vi "Message.vi"(8 "error in (no error)":errorcluster, 9 "Additional text":string, 10 "Message":T1) -> (0 "error out":errorcluster)   [LabVIEW 2013, in "Template-class-by-reference.lvlib" / "Template.lvclass"]
uses:
  Template.lvclass
  Messages.ctl
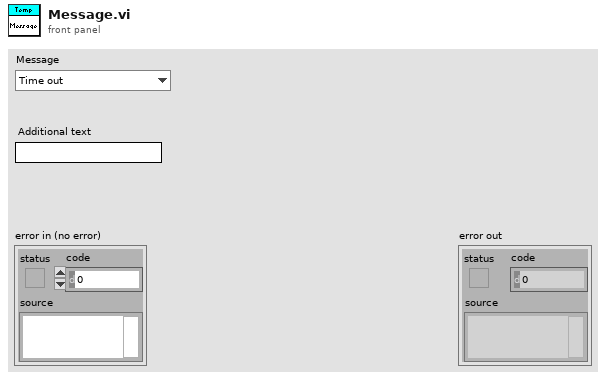
[diagram p1: front panel]
types:
  T1 = typedef "Template-class-by-reference.lvlib/Template.lvclass/Messages.ctl" = enum16{"Time out", "User cancel", "Module cancel"}
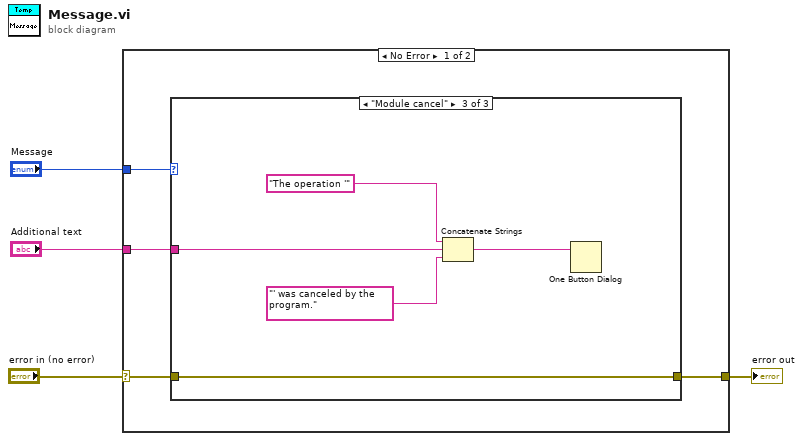
[diagram p0: block diagram]
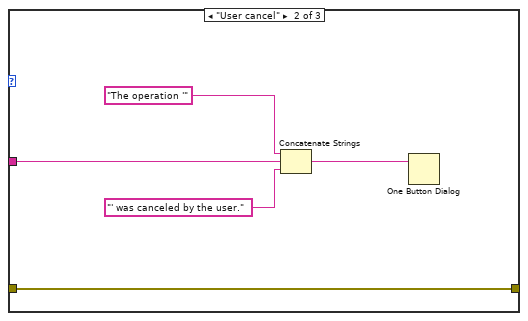
[diagram p3: hidden frame]
diagram:
  n1 = case shown="No Error" "error in (no error)" {
    selector: "error in (no error)" -> [w8 w20]
    tunnel: [w5 w20] -> w3
    tunnel: "Message" -> [w7 _]
    tunnel: "Additional text" -> [w6 _]
    frame No Error {
      n2 = case shown="\"Module cancel\"" w7 {
        tunnel: w8 -> [w9 w14 w19]
        tunnel: w6 -> [_ w13 w18]
        tunnel: [w9 w14 w19] -> w5
        frame Default {
        }
        frame "User cancel" {
          n3 = Concatenate Strings("The operation '", w13, "' was canceled by the user.") -> (w10:string)
          n4 = One Button Dialog(message=w10) -> ()  [unwired: 1 in, 1 out]
        }
        frame "Module cancel" {
          n5 = Concatenate Strings("The operation '", w18, "' was canceled by the program.") -> (w15:string)
          n6 = One Button Dialog(message=w15) -> ()  [unwired: 1 in, 1 out]
        }
      }
    }
    frame Error {
    }
  }
  "error out" <- w3
